vi "ReadData.vi"(8 "error in (no error)":errorcluster, 10 "Task":string, 11 "DAQ_Module in":refnum<class "DAQ_Module.lvclass">) -> (0 "error out":errorcluster, 2 "Waveform":waveform(dbl)[](array[waveform]), 3 "DAQ_Module out":refnum<class "DAQ_Module.lvclass">)   [LabVIEW 2025, in "DAQ_Module.lvlib" / "DAQ_Module.lvclass"]
uses:
  DAQ_Module.lvclass
  DAQ_Module.lvclass/DAQ_Module.ctl
  DAQ_Abstr/Task_Abstr/Task_Abstr Messages/ReadData Msg/ReadData Msg.lvclass/ReadData Msg.ctl
  <vilib>/ActorFramework/Message Enqueuer/Message Enqueuer.lvclass/Message Enqueuer.ctl
  <vilib>/ActorFramework/Message Enqueuer/Enqueue.vi
  DAQ_Abstr/Task_Abstr/Task_Abstr Messages/ReadData Msg/ReadData Msg.lvclass
  <vilib>/ActorFramework/Message Priority Queue/Priority Enqueue.vi
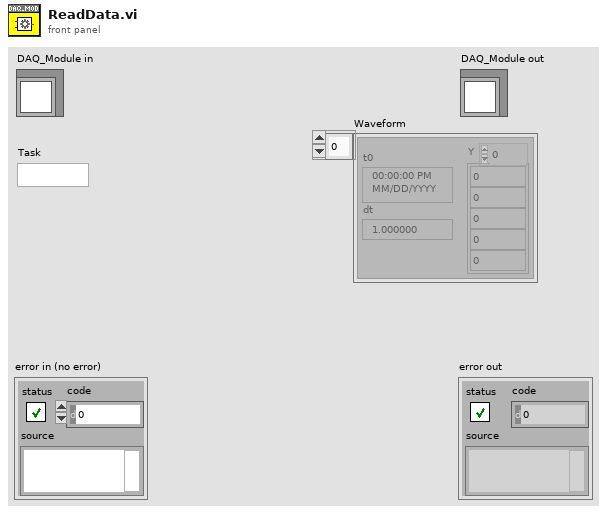
[diagram p1: front panel]
types:
  T1 = map{string, refnum<class "Message Enqueuer.lvclass">}
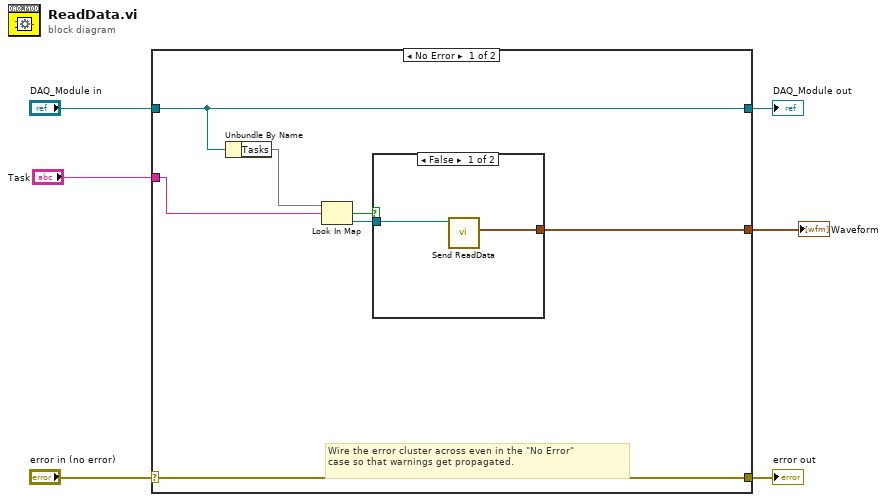
[diagram p0: block diagram]
diagram:
  n1 = case shown="No Error" "error in (no error)" {
    selector: "error in (no error)" -> [w13 w17]
    tunnel: [w13 w17] -> w5
    tunnel: [w9 w16] -> w3
    tunnel: "DAQ_Module in" -> [w9 w16]
    tunnel: "Task" -> [w8 _]
    tunnel: [w7 _] -> w1
    frame No Error {
      # "Wire the error cluster across even in the \"No Error\"\ncase so that warnings get propagated."
      n2 = Unbundle By Name(w9) -> ("Tasks"=w12:T1)
      n3 = Look In Map(map=w12, key=w8) -> (key not found?=w10:bool, value=w11:refnum<class "Message Enqueuer.lvclass">)  [unwired: 1 in]
      n4 = case shown="False" w10 {
        tunnel: w11 -> [w15 _]
        tunnel: [w14 _] -> w7
        frame False {
          n5 = call "Send ReadData.vi"("Message Enqueuer"=w15) -> ("Waveform"=w14:waveform(dbl)[])  [unwired: 8 in, 2 out]
        }
        frame True {
        }
      }
    }
    frame Error {
    }
  }
  "error out" <- w5
  "DAQ_Module out" <- w3
  "Waveform" <- w1
